vi "test9-ModuleCreatedDestroyed_Event.vi"(8 "error in (no error)":errorcluster, 11 "TestCase in":refnum<class "testcase-CSMGlobalLog.lvclass">) -> (0 "error out":errorcluster, 3 "TestCase out":refnum<class "testcase-CSMGlobalLog.lvclass">)   [LabVIEW 2017, in "testcase-CSMGlobalLog.lvclass"]
uses:
  testcase-CSMGlobalLog.lvclass
  testcase-CSMGlobalLog.lvclass/testcase-CSMGlobalLog.ctl
  src/user.lib/_NEVSTOP/Communicable State Machine(CSM)/_Support/Typedef/_CSM_GlobalLog_MSG.ctl
  src/user.lib/_NEVSTOP/Communicable State Machine(CSM)/_Support/Typedef/_CSM_Response Source Message.ctl
  src/user.lib/_NEVSTOP/Communicable State Machine(CSM)/_Support/Typedef/_CSM_GlobalLog_MSG_TYPE.ctl
  24a778c7-405f-47d7-a6be-afdb60495ae4.vi
  src/user.lib/_NEVSTOP/Communicable State Machine(CSM)/_Support/GlobalEvent/GEvt-Generate with Rule Check.vi
  src/user.lib/_NEVSTOP/Communicable State Machine(CSM)/AdvanceAPI/CSM - Convert Error to Argument.vi
  src/user.lib/_NEVSTOP/Communicable State Machine(CSM)/_Support/GlobalEvent/Cache-GEvt Refs.vi
  src/user.lib/_NEVSTOP/Communicable State Machine(CSM)/AdvanceAPI/CSM - Make String Arguments Safe.vi
  src/user.lib/_NEVSTOP/Communicable State Machine(CSM)/_Support/ChangeFlag/FlagInstance-GEvt Refs.vi
  src/user.lib/_NEVSTOP/Communicable State Machine(CSM)/AdvanceAPI/CSM - Keywords.vi
  src/user.lib/_NEVSTOP/Communicable State Machine(CSM)/_Support/ChangeFlag/ChangeFlag-Read.vi
  src/user.lib/_NEVSTOP/Communicable State Machine(CSM)/_Support/ChangeFlag/ChangeFlagDB.vi
  src/user.lib/_NEVSTOP/Communicable State Machine(CSM)/_Support/GlobalEvent/FGV-GlobalEventRef(lvlibp).vi
  src/user.lib/_NEVSTOP/Communicable State Machine(CSM)/_Support/GlobalEvent/FGV-GlobalEventQueues(lvlibp).vi
  src/user.lib/_NEVSTOP/Communicable State Machine(CSM)/_Support/GlobalEvent/GEvt-Valid Subscribers.vi
  src/user.lib/_NEVSTOP/Communicable State Machine(CSM)/_Support/GlobalEvent/LogFilter/LogFilter - Check.vi
  src/user.lib/_NEVSTOP/Communicable State Machine(CSM)/_Support/GlobalEvent/LogFilter/LogFilter.lvclass
  <vilib>/addons/_JKI Toolkits/VI Tester/TestCase.llb/TestCase.lvclass
  src/user.lib/_NEVSTOP/Communicable State Machine(CSM)/Communicable State Machine.lvlib
  CSM/CSM-Testcase.lvlib
  C:/Program Files (x86)/National Instruments/LabVIEW 2017/vi.lib/addons/_JKI Toolkits/VI Tester/TestCase.llb/TestCase.lvclass
panel:
  out "String Cache Each Loop":string
  out "LoopCount":i32
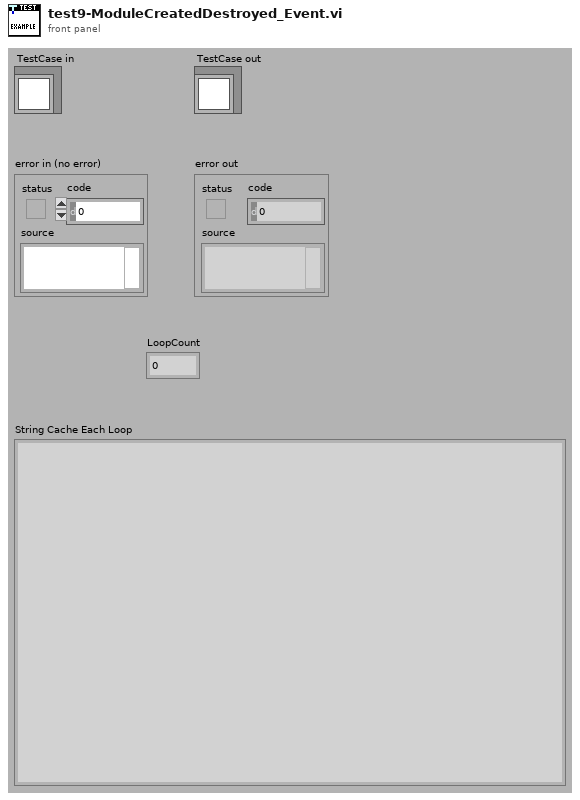
[diagram p1: front panel]
types:
  T1 = typedef "Communicable State Machine.lvlib/_CSM_GlobalLog_MSG.ctl" = cluster{"Name (\"\" to Use UUID)":string, "Current State":string, "Arguments":string, "Source Message":T2, "Source Module":string, "Complete(T)/Start(F)":bool, "LogType":T3, "Time Stamp":timestamp}
  T2 = typedef "Communicable State Machine.lvlib/_CSM_Response Source Message.ctl" = cluster{"‘State":string, "’Arguments":string, "’Error":errorcluster}
  T3 = typedef "Communicable State Machine.lvlib/_CSM_GlobalLog_MSG_TYPE.ctl" = enum16{"User Log", "State Change", "Status", "Interrupt", "Register", "Unregister", "Error Log", "Module Created", "Module Destroyed", "Async Message", "No-Rep Async Message", "Sync Message"}
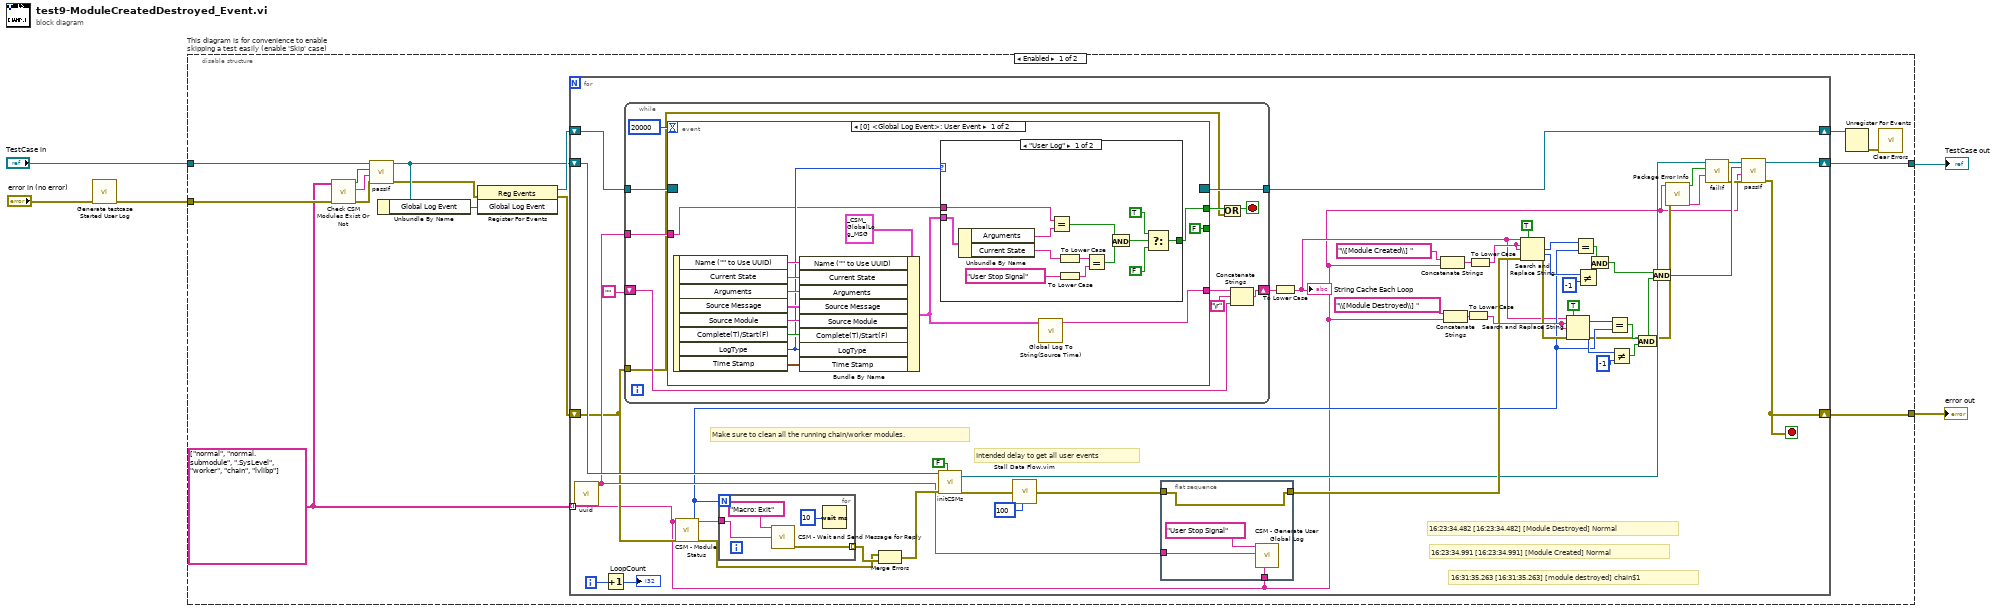
[diagram p0: block diagram]
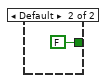
[diagram p2: hidden frame]
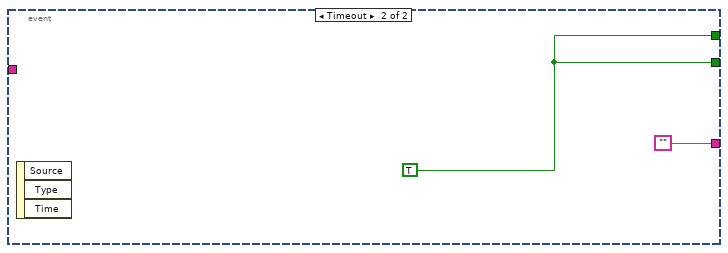
[diagram p3: hidden frame]
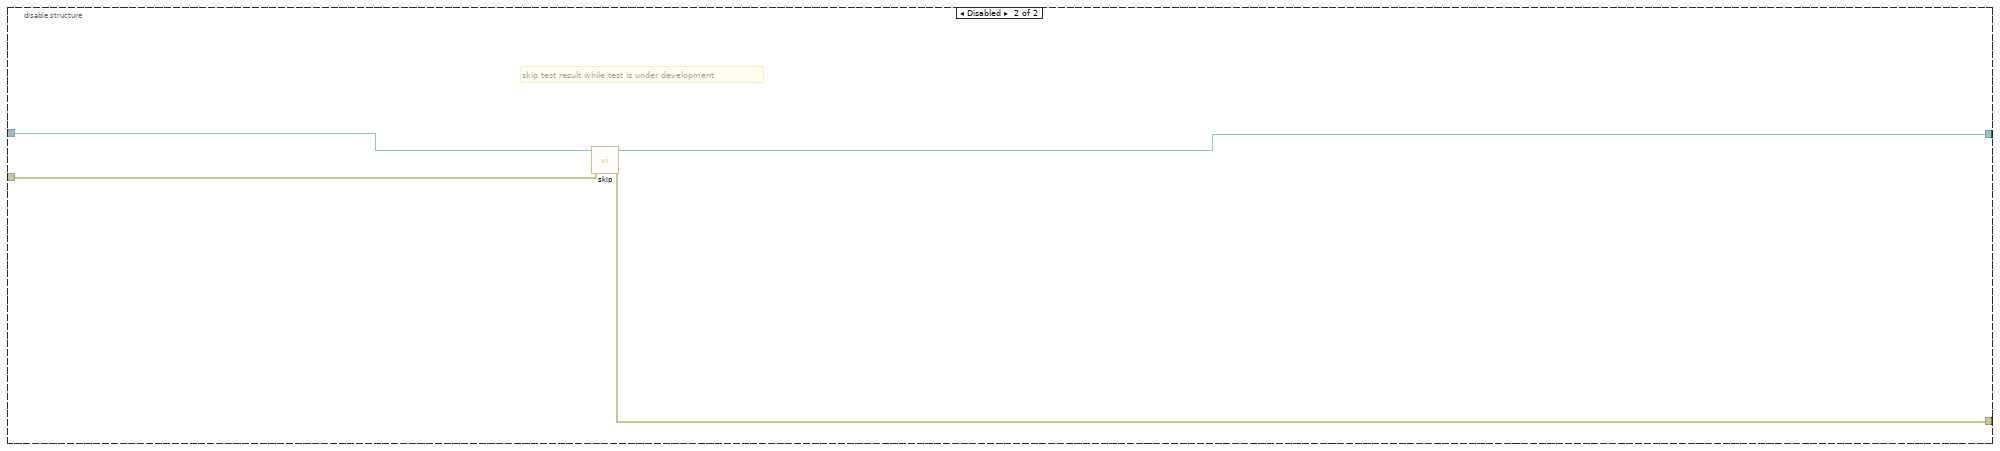
[diagram p4: hidden frame]
diagram:
  n1 = call "Generate testcase Started User Log.vi"("Error In"="error in (no error)") -> ("error out"=w1:errorcluster)  [unwired: 10 in]
  n2 = disable-structure "This diagram is for convenience to enable skipping a test easily (enable 'Skip' case)" shown="Enabled" {
    disable-tunnel: "TestCase in" -> [w11 w124]
    disable-tunnel: [w16 w122] -> w2
    disable-tunnel: [w15 w123] -> w4
    disable-tunnel: w1 -> [w9 w121]
    frame Enabled {
      w8 = string[] ["normal", "normal.submodule", ".SysLevel", "worker", "chain", "lvlibp"]
      n3 = call "Check CSM Modules Exist Or Not.vi"("error in"=w9, "CSM names in"=w8) -> ("error out"=w12:errorcluster, "Debug string"=w13:string, "All Modules Exist?"=w14:bool)  [unwired: 7 in]
      n4 = call-dynamic "passIf.vi"("error in (no error)"=w12, "message (\"\")"=w13, "pass"=w14, "TestCase in"=w11) -> ("error out"=w7:errorcluster, "TestCase out"=w10:refnum<class "testcase-CSMGlobalLog.lvclass">)  [unwired: 6 in]
      n5 = Unbundle By Name(w10) -> ("Global Log Event"=w20:refnum<user-event>)
      n6 = register-events(error in=w7, w20) -> (reference out=w19:refnum<event-registration>, error out=w17:errorcluster)  [unwired: 1 in]
      n7 = for {
        shift-right: [w70] -> w18
        shift-left: w19 -> [w71]
        shift-right: [w60] -> w15
        shift-left: w17 -> [w28]
        tunnel: w8 -> [w21] mode=indexing
        shift-right: [w63] -> w16
        shift-left: w10 -> [w64]
        i -> [w62]
        stop <- w60 stop-if-true
        # "16:31:35.263 [16:31:35.263] [module destroyed] chain$1"
        # "16:23:34.991 [16:23:34.991] [Module Created] Normal"
        # "16:23:34.482 [16:23:34.482] [Module Destroyed] Normal"
        # "Intended delay to get all user events"
        # "Make sure to clean all the running chain/worker modules."
        n8 = call "uuid.vi"() -> ("UUID"=w59:string)  [unwired: 11 in]
        n9 = Increment(x=w62) -> (x+1=→"LoopCount":i32)
        n10 = while {
          tunnel: w71 -> [w90]
          tunnel: [w89] -> w70
          shift-right: [w82] -> w31
          shift-left: "" -> [w83]
          tunnel: w59 -> [w86]
          tunnel: w28 -> [w80]
          stop <- w81 stop-if-true
          n11 = event shown="[0] <Global Log Event>: User Event" {
            selector: w90 -> [_ _]
            dyn-events: [_ _] -> w89
            timeout: 20000 -> [_ _]
            tunnel: [w96 ""] -> w85
            tunnel: [w91 w120] -> w88
            tunnel: w86 -> [w92 _]
            tunnel: [FALSE ("Stop") w120] -> _
            event User Event {
              n12 = event-data() -> ("Name (\"\" to Use UUID)"=w103:string, "Current State"=w102:string, "Arguments"=w101:string, "Source Message"=w100:T2, "Source Module"=w99:string, "Complete(T)/Start(F)"=w98:bool, "LogType"=w94:T3, "Time Stamp"=w97:timestamp)  [unwired: 1 in]
              n13 = Bundle By Name(cluster=T1 {"Name (\"\" to Use UUID)"="", "Current State"="", "Arguments"="", "Source Message"={"‘State"="", "’Arguments"="", "’Error"={"status"=FALSE, "code"=0, "source"=""}}, "Source Module"="", "Complete(T)/Start(F)"=FALSE, "LogType"=enum."State Change", "Time Stamp"=timestamp(0 s since 1904-01-01)} ("Cross CSM Data"), "Name (\"\" to Use UUID)"=w103, "Current State"=w102, "Arguments"=w101, "Source Message"=w100, "Source Module"=w99, "Complete(T)/Start(F)"=w98, "LogType"=w94, "Time Stamp"=w97) -> (w93:T1)
              n14 = case shown="\"User Log\"" w94 {
                tunnel: w93 -> [w117 _]
                tunnel: w92 -> [w116 _]
                tunnel: [w105 FALSE] -> w91
                frame "User Log" {
                  n15 = Unbundle By Name(w117) -> ("Arguments"=w115:string, "Current State"=w114:string)
                  n16 = Equal?(x=w116, y=w115) -> (x = y?=w109:bool)
                  n17 = To Lower Case(string=w114) -> (all lower case string=w113:string)
                  n18 = To Lower Case(string="User Stop Signal" ("Log")) -> (all lower case string=w111:string)
                  n19 = Equal?(x=w113, y=w111) -> (x = y?=w110:bool)
                  n20 = And(x=w109, y=w110) -> (x .and. y?=w108:bool)
                  n21 = Select(t=TRUE, s=w108, f=FALSE) -> (s? t:f=w105:bool)
                }
                frame Default {
                }
              }
              n22 = call "Global Log To String(Source Time).vi"("Log"=w93) -> ("Log String"=w96:string)  [unwired: 9 in]
            }
            event Timeout {
              w120 = TRUE ("Stop")
              n23 = event-data() -> ()  [unwired: 1 in, 3 out]
            }
          }
          n24 = Or(x=w88, y=w80) -> (x .or. y?=w81:bool)
          n25 = Concatenate Strings(w85, "\r", w83) -> (w82:string)
        }
        n26 = call "CSM - Module Status.vi"("Error In"=w28, "CSM Name"=w21) -> ("error out"=w67:errorcluster, "#Nodes"=w33:i32, "CSM Name (Dup)"=w69:string)  [unwired: 5 in, 2 out]
        n27 = for {
          N: w33 -> [_]
          tunnel: [w78] -> w68 mode=indexing
          tunnel: w69 -> [w77]
          n28 = call "CSM - Wait and Send Message for Reply.vi"("State"="Macro: Exit", "Target Module"=w77) -> ("error out"=w78:errorcluster)  [unwired: 10 in, 3 out]
          n29 = Wait (ms)(milliseconds to wait=u32 10) -> ()  [unwired: 1 out]
        }
        n30 = Merge Errors(w67, w68) -> (w66:errorcluster)
        n31 = call "initCSMs.vi"("Enable building lvlibp?"=FALSE, "error in (no error)"=w66, "TestCase in"=w64) -> ("error out"=w57:errorcluster, "TestCase out"=w26:refnum<class "testcase-CSMGlobalLog.lvclass">)  [unwired: 7 in]
        n32 = call "Stall Data Flow.vim"("value in"=w57, "milliseconds to wait"=u32 100) -> ("value out"=w56:errorcluster)  [unwired: 1 out]
        n33 = flat-sequence {
          tunnel: w56 -> [w72]
          tunnel: [w72] -> w34
          tunnel: w59 -> [w74]
          tunnel: w21 -> [w73]
          frame #0 {
            n34 = call "CSM - Generate User Global Log.vi"("From Who"=w73, "Arguments"=w74, "Log"="User Stop Signal") -> ()  [unwired: 8 in, 1 out]
          }
        }
        n35 = To Lower Case(string=w31) -> (all lower case string=w30:string)
        "String Cache Each Loop" <- w30
        n36 = Concatenate Strings("\\[Module Created\\] " ("regular expression"), w21) -> (w52:string)
        n37 = Concatenate Strings("\\[Module Destroyed\\] " ("regular expression"), w21) -> (w54:string)
        n38 = To Lower Case(string=w54) -> (all lower case string=w38:string)
        n39 = To Lower Case(string=w52) -> (all lower case string=w50:string)
        n40 = Search and Replace String(replace all?=TRUE ("replace all? (F)"), input string=w30, search string=w50, replace string=w50, error in=w34) -> (number of replacements=w49:i32, offset past replacement=w48:i32, error out=w37:errorcluster)  [unwired: 3 in, 1 out]
        n41 = Search and Replace String(replace all?=TRUE ("replace all? (F)"), input string=w30, search string=w38, replace string=w38, error in=w37) -> (number of replacements=w40:i32, offset past replacement=w41:i32, error out=w22:errorcluster)  [unwired: 3 in, 1 out]
        n42 = Equal?(x=w49, y=w33) -> (x = y?=w46:bool)
        n43 = Not Equal?(x=w48, y=-1) -> (x != y?=w45:bool)
        n44 = And(x=w46, y=w45) -> (x .and. y?=w36:bool)
        n45 = Equal?(x=w40, y=w33) -> (x = y?=w43:bool)
        n46 = Not Equal?(x=w41, y=-1) -> (x != y?=w44:bool)
        n47 = And(x=w43, y=w44) -> (x .and. y?=w35:bool)
        n48 = And(x=w36, y=w35) -> (x .and. y?=w32:bool)
        n49 = call "Package Error Info.vi"("error in"=w22, "String in"=w21) -> ("packed error info out"=w23:string, "error status"=w27:bool)  [unwired: 8 in]
        n50 = call-dynamic "failIf.vi"("message (\"\")"=w23, "fail"=w27, "TestCase in"=w26) -> ("error out"=w24:errorcluster, "TestCase out"=w25:refnum<class "testcase-CSMGlobalLog.lvclass">)  [unwired: 7 in]
        n51 = call-dynamic "passIf.vi"("error in (no error)"=w24, "message (\"\")"=w21, "pass"=w32, "TestCase in"=w25) -> ("error out"=w60:errorcluster, "TestCase out"=w63:refnum<class "testcase-CSMGlobalLog.lvclass">)  [unwired: 6 in]
      }
      n52 = Unregister For Events(event registration refnum=w18) -> (error out=w6:errorcluster)  [unwired: 1 in]
      n53 = call <vilib>:"Clear Errors.vi"("error in (no error)"=w6) -> ()  [unwired: 5 in, 2 out]
    }
    frame Disabled {
      # "skip test result while test is under development"
      n54 = call <vilib>:"skip.vi"("error in (no error)"=w121, "TestCase in"=w124) -> ("error out"=w123:errorcluster, "TestCase out"=w122:refnum<class "testcase-CSMGlobalLog.lvclass">)  [unwired: 8 in]
    }
  }
  "error out" <- w4
  "TestCase out" <- w2
